vi "prosess_data.vi"(0 "Q_MotorCmd_IN":refnum<queue>, 1 "Q_MotorCmd_Err_IN":errorcluster, 2 "Q_Process_Data_IN":refnum<queue>, 3 "Q_Process_Data_Err_IN":errorcluster caption="Q_Process_DATA_Err_IN", 4 "Notifier_IN":refnum<notifier>, 5 "Error_IN":errorcluster caption="Notifier Error IN", 6 "Q_DATA_IN":refnum<queue>, 8 "Q_DATA_Err_IN":errorcluster) -> (14 "Q_Process_Data_OUT":refnum<queue>, 15 "Q_Process_Data_Err_OUT":errorcluster caption="Q_Process_DATA_Err_OUT", 16 "Q_MotorCmd_OUT":refnum<queue>, 17 "Q_MotorCmd_Err_OUT":errorcluster)   [LabVIEW 2019]
uses:
  <vilib>/Platform/TimedLoop/XDataNode/timing_clust.ctl
  <vilib>/Platform/TimedLoop/XDataNode/nitl_modes.ctl
  <vilib>/Platform/TimedLoop/XDataNode/wakeup.ctl
  RT_GLOBAL.vi
  <vilib>/Platform/TimedLoop/XDataNode/XDataNode.xnode
  <vilib>/Platform/TimedLoop/XDataNode/XDNodeRunTimeDep.lvlib
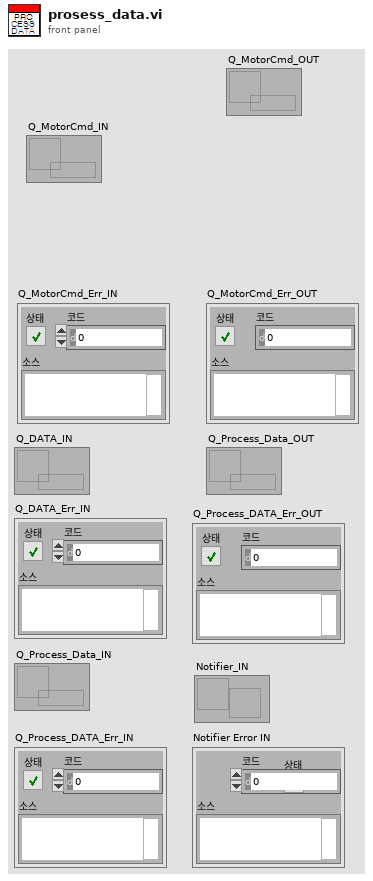
[diagram p1: front panel]
types:
  T1 = cluster{"MinPos":i32, "MaxPos":i32, "Init_Vel_UP":i32, "Init_Accel":u32, "Test_Vel":i32, "Test_Acc":u32, "Init_Onset_Load":sgl, "Init_L":bool, "Init_R":bool, "Param":cluster{"Clt_Param_L":cluster{"기준값":sgl, "검출값":sgl, "Onset_Min":sgl, "Onset_Max":sgl, "Peak_Min":sgl, "Peak_Max":sgl, "Base":i32, "Onset":i32, "Peak":i32, "Pos":i32, "Offset":sgl}, "Clt_Param_R":cluster{"기준값":sgl, "검출값":sgl, "Onset_Min":sgl, "Onset_Max":sgl, "Peak_Min":sgl, "Peak_Max":sgl, "Base":i32, "Onset":i32, "Peak":i32, "Pos":i32, "Offset":sgl}}, "Onset_Load_L":sgl, "Max_Load_L":sgl, "Onset_Load_R":sgl, "Max_Load_R":sgl, "Init_Vel_DWON":i32, "Load_Warn":sgl, "Load_Alarm":sgl}
  T2 = typedef "XDNodeRunTimeDep.lvlib/timing_clust.ctl" = cluster{"Expected End [f-1]":u64, "Actual End [f-1]":u64, "Finished Late? [f-1]":bool, "Expected End [i-1]":u64, "Actual End [i-1]":u64, "Finished Late? [i-1]":bool, "Expected Start [i]":u64, "Actual Start [i]":u64, "Expected Start [f]":u64, "Actual Start [f]":u64, "Source Name":string, "Structure Name":string, "Period":i64, "Deadline":i64, "Offset":i64, "Start":i64, "Priority":i32, "Timeout":i32, "Mode":T3, "Wakeup Reason":T4, "Error":errorcluster, "Source Type":string, "Secondary Source Type":string, "Global End Time":u64, "Global Start Time":u64, "Frame Duration":u64, "Iteration Duration":u64, "Assigned CPU":i32, "I/O Scan Engine Mode":u32}
  T3 = typedef "XDNodeRunTimeDep.lvlib/nitl_modes.ctl" = enum32{"No Change", "Process missed periods, maintain original phase", "Discard missed periods, maintain original phase", "Process missed periods, ignore original phase", "Discard missed periods, ignore original phase"}
  T4 = typedef "XDNodeRunTimeDep.lvlib/wakeup.ctl" = enum32{"Normal", "Aborted", "Asynchronous wakeup", "Timing source error", "Timed loop error", "Timeout"}
  T5 = cluster{"Num_L":u32, "Period_L":u32, "GCP_L":sgl, "Num_R":u32, "Period_R":u32, "GCP_R":sgl, "FPGA_Data":sgl[], "Status_L":cluster{"Ready to switch on":bool, "Switched on":bool, "Operation enable":bool, "Fault":bool, "Voltage enable":bool, "Quick stop":bool, "Switch on disable":bool, "not used (warning)":bool, "Offset current measured":bool, "Remote":bool, "Operation mode specific":bool, "Internal limit active":bool, "Operation mode specific":bool, "Operation mode specific":bool, "Refresh cycle of power stage":bool, "Position referenced to home position":bool}, "Status_R":cluster{"Ready to switch on":bool, "Switched on":bool, "Operation enable":bool, "Fault":bool, "Voltage enable":bool, "Quick stop":bool, "Switch on disable":bool, "not used (warning)":bool, "Offset current measured":bool, "Remote":bool, "Operation mode specific":bool, "Internal limit active":bool, "Operation mode specific":bool, "Operation mode specific":bool, "Refresh cycle of power stage":bool, "Position referenced to home position":bool}, "Pos_L":i32, "Pos_R":i32, "TargetPos_L":i32, "TargetPos_R":i32, "Flag_L":enum16{"Release_Start", "Onset_Start", "Peak_Start", "Calculate"}, "Flag_R":enum16{"Release_Start", "Onset_Start", "Peak_Start", "Calculate"}, "LOAD_CELL_PEAK_L":sgl[], "LOAD_CELL_PEAK_R":sgl[], "D_Pos_L":i32, "D_Pos_R":i32, "A_Velocity_L":i32, "A_Velocity_R":i32, "A_Current_L":i16, "A_Current_R":i16}
  T6 = cluster{"Cmd":string, "Data1":variant, "Data2":variant}
  T7 = cluster{"FPGA_Data":sgl[], "Tick":u32, "Cmd":string, "Param":variant}
  T8 = cluster{"Ready to switch on":bool, "Switched on":bool, "Operation enable":bool, "Fault":bool, "Voltage enable":bool, "Quick stop":bool, "Switch on disable":bool, "not used (warning)":bool, "Offset current measured":bool, "Remote":bool, "Operation mode specific":bool, "Internal limit active":bool, "Operation mode specific":bool, "Operation mode specific":bool, "Refresh cycle of power stage":bool, "Position referenced to home position":bool}
  T9 = enum16{"Release_Start", "Onset_Start", "Peak_Start", "Calculate"}
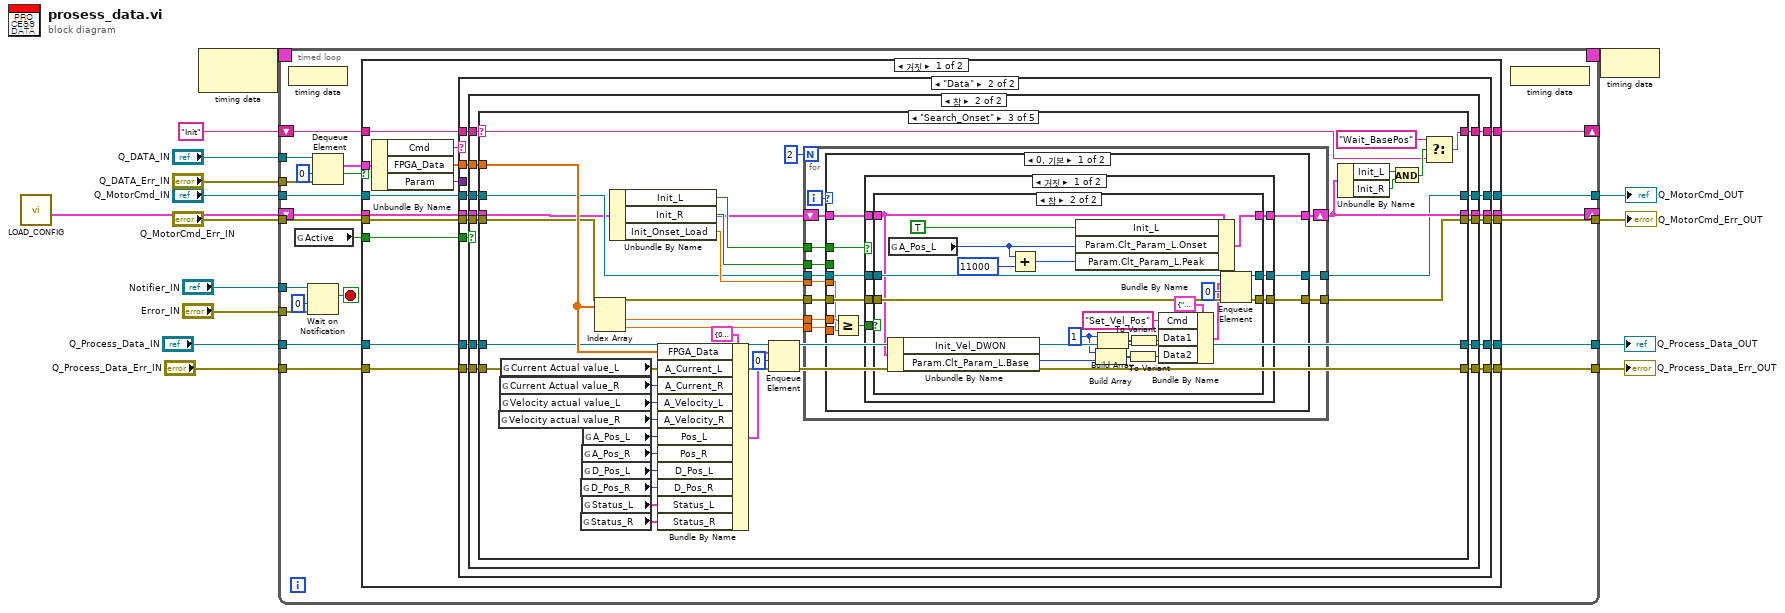
[diagram p0: block diagram]
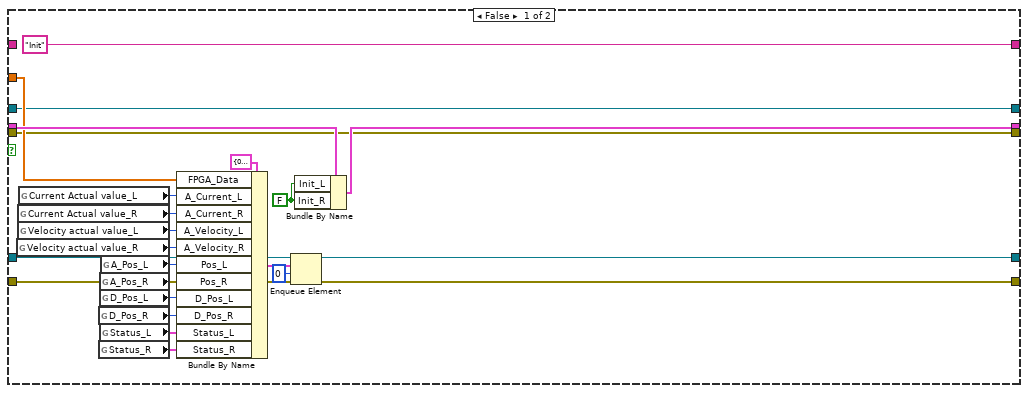
[diagram p3: hidden frame]
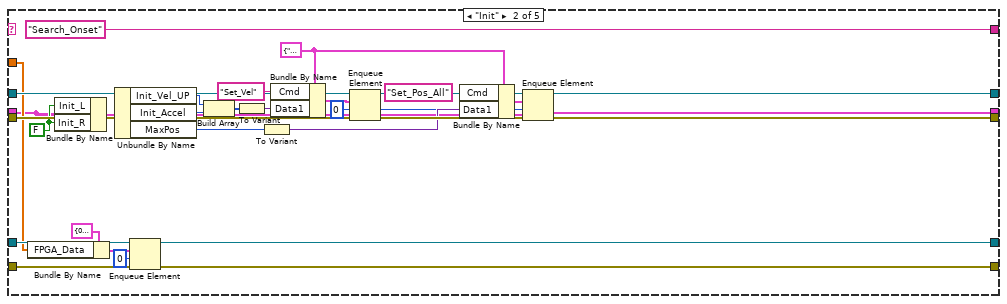
[diagram p5: hidden frame]
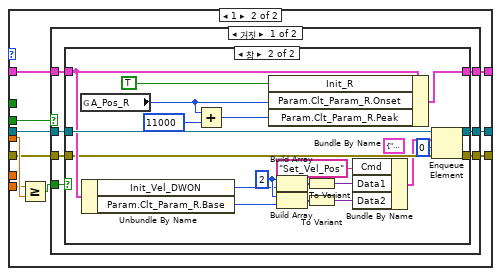
[diagram p8: hidden frame]
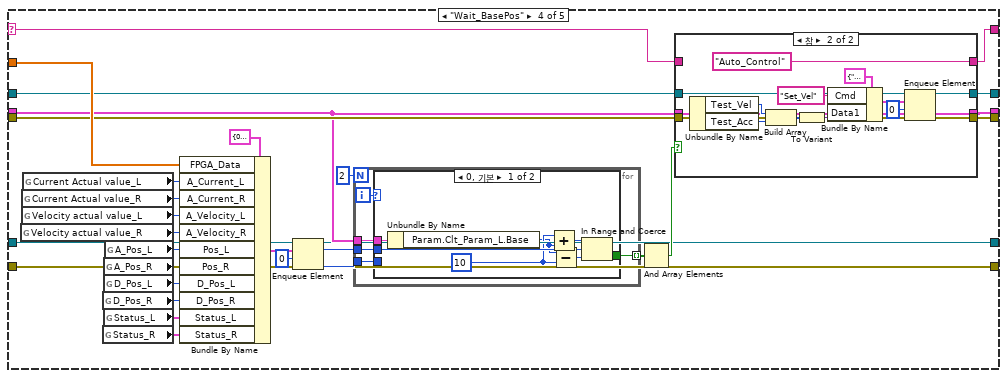
[diagram p11: hidden frame]
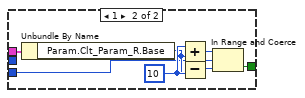
[diagram p13: hidden frame]
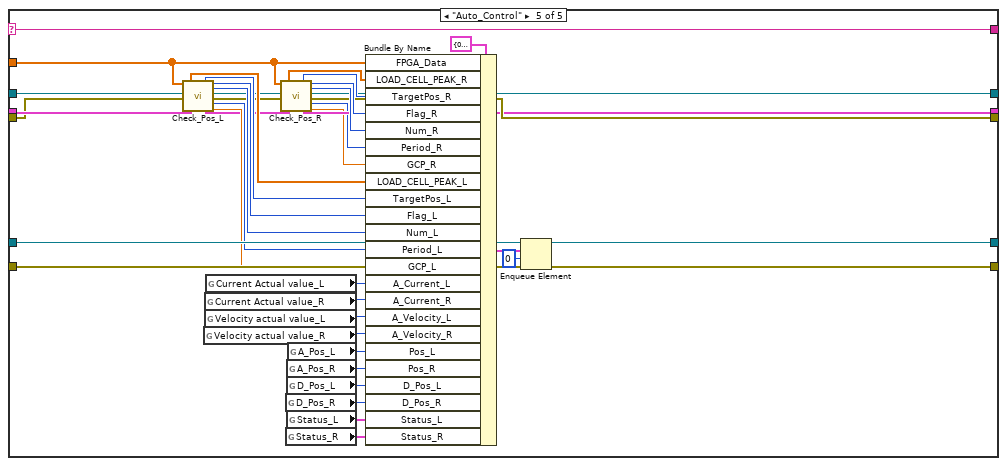
[diagram p14: hidden frame]
diagram:
  n1 = call "LOAD_CONFIG.vi"() -> ("Param_Out"=w7:T1)  [unwired: 10 in, 1 out]
  n2 = node-c288() -> (w9:T2)  [unwired: 1 in]
  n3 = timed-loop {
    shift-right: [w37] -> _
    shift-left: "Init" -> [w38]
    tunnel: "Q_DATA_IN" -> [w35]
    tunnel: "Q_DATA_Err_IN" -> [w34]
    tunnel: "Q_MotorCmd_IN" -> [w30]
    tunnel: "Q_MotorCmd_Err_IN" -> [w29]
    tunnel: "Q_Process_Data_IN" -> [w28]
    tunnel: "Q_Process_Data_Err_IN" -> [w27]
    timing: w9 -> [_]
    timing-out: [_] -> w8
    shift-right: [w25] -> _
    shift-left: w7 -> [w26]
    tunnel: "Notifier_IN" -> [w22]
    tunnel: "Error_IN" -> [w21]
    tunnel: [w20] -> w4
    tunnel: [w19] -> w3
    tunnel: [w18] -> w2
    tunnel: [w17] -> w1
    stop <- w24 stop-if-true
    n4 = node-c288() -> ()  [unwired: 1 in]
    n5 = global read "RT_GLOBAL.vi" "Active"() -> (w31:bool)
    n6 = Wait on Notification(notifier=w22, timeout in ms (-1)=0 ("타임아웃(ms) (-1)"), error in (no error)=w21) -> (notification=w24:bool)  [unwired: 1 in, 3 out]
    n7 = Dequeue Element(queue=w35, timeout in ms (-1)=0 ("타임아웃(ms) (-1)"), error in (no error)=w34) -> (element=w32:T7, timed out?=w33:bool)  [unwired: 2 out]
    n8 = case shown="거짓" w33 {
      tunnel: [w47 w398] -> w25
      tunnel: w26 -> [w54 w398]
      tunnel: w38 -> [w57 w397]
      tunnel: [w50 w397] -> w37
      tunnel: w32 -> [w56 _]
      tunnel: w31 -> [w51 _]
      tunnel: w30 -> [w49 w396]
      tunnel: w29 -> [w48 w395]
      tunnel: w28 -> [w46 w394]
      tunnel: w27 -> [w45 w393]
      tunnel: [w44 w396] -> w20
      tunnel: [w43 w395] -> w19
      tunnel: [w42 w394] -> w18
      tunnel: [w41 w393] -> w17
      frame False {
        n9 = Unbundle By Name(w56) -> ("Cmd"=w55:string, "FPGA_Data"=w52:sgl[], "Param"=w53:variant)
        n10 = case shown="\"Data\"" w55 {
          tunnel: w57 -> [w63 w77]
          tunnel: w54 -> [w62 w75]
          tunnel: w53 -> [_ _]
          tunnel: w52 -> [_ w76]
          tunnel: w51 -> [_ w74]
          tunnel: [w63 w73] -> w50
          tunnel: w49 -> [w61 w72]
          tunnel: w48 -> [w60 w71]
          tunnel: [w62 w70] -> w47
          tunnel: w46 -> [w59 w69]
          tunnel: w45 -> [w58 w68]
          tunnel: [w61 w67] -> w44
          tunnel: [w60 w66] -> w43
          tunnel: [w59 w65] -> w42
          tunnel: [w58 w64] -> w41
          frame "거짓", Default {
          }
          frame "Data" {
            n11 = case shown="참" w74 {
              tunnel: w77 -> [_ w107]
              tunnel: w76 -> [w93 w110]
              tunnel: w75 -> [w99 w113]
              tunnel: ["Init" w114] -> w73
              tunnel: w72 -> [w81 w112]
              tunnel: w71 -> [w80 w111]
              tunnel: [w98 w109] -> w70
              tunnel: w69 -> [w95 w108]
              tunnel: w68 -> [w94 w106]
              tunnel: [w81 w105] -> w67
              tunnel: [w80 w104] -> w66
              tunnel: [w79 w103] -> w65
              tunnel: [w78 w102] -> w64
              frame False {
                w100 = FALSE ("Init_L")
                n12 = global read "RT_GLOBAL.vi" "Velocity actual value_R"() -> (w88:i32)
                n13 = global read "RT_GLOBAL.vi" "Current Actual value_R"() -> (w90:i16)
                n14 = global read "RT_GLOBAL.vi" "Velocity actual value_L"() -> (w89:i32)
                n15 = global read "RT_GLOBAL.vi" "Current Actual value_L"() -> (w91:i16)
                n16 = global read "RT_GLOBAL.vi" "D_Pos_R"() -> (w84:i32)
                n17 = global read "RT_GLOBAL.vi" "Status_R"() -> (w82:T8)
                n18 = global read "RT_GLOBAL.vi" "A_Pos_R"() -> (w86:i32)
                n19 = global read "RT_GLOBAL.vi" "D_Pos_L"() -> (w85:i32)
                n20 = global read "RT_GLOBAL.vi" "Status_L"() -> (w83:T8)
                n21 = global read "RT_GLOBAL.vi" "A_Pos_L"() -> (w87:i32)
                n22 = Bundle By Name(cluster=T5 {"Num_L"=0, "Period_L"=0, "GCP_L"=0.0, "Num_R"=0, "Period_R"=0, "GCP_R"=0.0, "FPGA_Data"=[], "Status_L"={"Ready to switch on"=TRUE, "Switched on"=TRUE, "Operation enable"=TRUE, "Fault"=FALSE, "Voltage enable"=TRUE, "Quick stop"=TRUE, "Switch on disable"=FALSE, "not used (warning)"=FALSE, "Offset current measured"=FALSE, "Remote"=TRUE, "Operation mode specific"=TRUE, "Internal limit active"=FALSE, "Operation mode specific"=FALSE, "Operation mode specific"=FALSE, "Refresh cycle of power stage"=FALSE, "Position referenced to home position"=FALSE}, "Status_R"={"Ready to switch on"=TRUE, "Switched on"=TRUE, "Operation enable"=TRUE, "Fault"=FALSE, "Voltage enable"=TRUE, "Quick stop"=TRUE, "Switch on disable"=FALSE, "not used (warning)"=FALSE, "Offset current measured"=FALSE, "Remote"=TRUE, "Operation mode specific"=TRUE, "Internal limit active"=FALSE, "Operation mode specific"=FALSE, "Operation mode specific"=FALSE, "Refresh cycle of power stage"=FALSE, "Position referenced to home position"=FALSE}, "Pos_L"=0, "Pos_R"=0, "TargetPos_L"=0, "TargetPos_R"=0, "Flag_L"=enum."Release_Start", "Flag_R"=enum."Release_Start", "LOAD_CELL_PEAK_L"=[12.0, 8.0], "LOAD_CELL_PEAK_R"=[], "D_Pos_L"=0, "D_Pos_R"=0, "A_Velocity_L"=0, "A_Velocity_R"=0, "A_Current_L"=0, "A_Current_R"=0}, "FPGA_Data"=w93, "A_Current_L"=w91, "A_Current_R"=w90, "A_Velocity_L"=w89, "A_Velocity_R"=w88, "Pos_L"=w87, "Pos_R"=w86, "D_Pos_L"=w85, "D_Pos_R"=w84, "Status_L"=w83, "Status_R"=w82) -> (w97:T5)
                n23 = Enqueue Element(queue=w95, element=w97, timeout in ms (-1)=0 ("타임아웃(ms) (-1)"), error in (no error)=w94) -> (queue out=w79:refnum<queue>, error out=w78:errorcluster)  [unwired: 1 out]
                n24 = Bundle By Name(cluster=w99, "Init_L"=w100, "Init_R"=w100) -> (w98:T1)
              }
              frame True {
                n25 = case shown="\"Search_Onset\"" w107 {
                  selector: w107 -> [w120 _ w172 w297 w389]
                  tunnel: [w120 "Search_Onset" w173 w292 w389] -> w114
                  tunnel: w113 -> [w119 w128 w155 w293 w373]
                  tunnel: w112 -> [w118 w149 w170 w294 w368]
                  tunnel: w111 -> [w117 w148 w169 w295 w369]
                  tunnel: w110 -> [_ w143 w182 w314 w365]
                  tunnel: [w119 w129 w171 w287 w357] -> w109
                  tunnel: w108 -> [w116 w145 w180 w311 w391]
                  tunnel: w106 -> [w115 w144 w179 w310 w388]
                  tunnel: [w118 w124 w154 w291 w360] -> w105
                  tunnel: [w117 w123 w153 w290 w359] -> w104
                  tunnel: [w116 w122 w152 w289 w354] -> w103
                  tunnel: [w115 w121 w151 w288 w353] -> w102
                  frame "거짓", Default {
                  }
                  frame "Init" {
                    w133 = T6 {"Cmd"="", "Data1"=variant, "Data2"=variant}
                    w134 = FALSE ("Init_L")
                    w130 = 0 ("타임아웃(ms) (-1)")
                    n26 = Bundle By Name(cluster=T5 {"Num_L"=0, "Period_L"=0, "GCP_L"=0.0, "Num_R"=0, "Period_R"=0, "GCP_R"=0.0, "FPGA_Data"=[], "Status_L"={"Ready to switch on"=TRUE, "Switched on"=TRUE, "Operation enable"=TRUE, "Fault"=FALSE, "Voltage enable"=TRUE, "Quick stop"=TRUE, "Switch on disable"=FALSE, "not used (warning)"=FALSE, "Offset current measured"=FALSE, "Remote"=TRUE, "Operation mode specific"=TRUE, "Internal limit active"=FALSE, "Operation mode specific"=FALSE, "Operation mode specific"=FALSE, "Refresh cycle of power stage"=FALSE, "Position referenced to home position"=FALSE}, "Status_R"={"Ready to switch on"=TRUE, "Switched on"=TRUE, "Operation enable"=TRUE, "Fault"=FALSE, "Voltage enable"=TRUE, "Quick stop"=TRUE, "Switch on disable"=FALSE, "not used (warning)"=FALSE, "Offset current measured"=FALSE, "Remote"=TRUE, "Operation mode specific"=TRUE, "Internal limit active"=FALSE, "Operation mode specific"=FALSE, "Operation mode specific"=FALSE, "Refresh cycle of power stage"=FALSE, "Position referenced to home position"=FALSE}, "Pos_L"=0, "Pos_R"=0, "TargetPos_L"=0, "TargetPos_R"=0, "Flag_L"=enum."Release_Start", "Flag_R"=enum."Release_Start", "LOAD_CELL_PEAK_L"=[12.0, 8.0], "LOAD_CELL_PEAK_R"=[], "D_Pos_L"=0, "D_Pos_R"=0, "A_Velocity_L"=0, "A_Velocity_R"=0, "A_Current_L"=0, "A_Current_R"=0}, "FPGA_Data"=w143) -> (w147:T5)
                    n27 = Bundle By Name(cluster=w128, "Init_L"=w134, "Init_R"=w134) -> (w129:T1)
                    n28 = Unbundle By Name(w128) -> ("Init_Vel_UP"=w127:i32, "Init_Accel"=w126:u32, "MaxPos"=w125:i32)
                    n29 = Enqueue Element(queue=w145, element=w147, timeout in ms (-1)=0 ("타임아웃(ms) (-1)"), error in (no error)=w144) -> (queue out=w122:refnum<queue>, error out=w121:errorcluster)  [unwired: 1 out]
                    n30 = Build Array(w127, w126) -> (w139:u32[])
                    n31 = To Variant(anything=w139) -> (Variant=w140:variant)
                    n32 = To Variant(anything=w125) -> (Variant=w135:variant)
                    n33 = Bundle By Name(cluster=w133, "Cmd"="Set_Vel", "Data1"=w140) -> (w132:T6)
                    n34 = Enqueue Element(queue=w149, element=w132, timeout in ms (-1)=w130, error in (no error)=w148) -> (queue out=w138:refnum<queue>, error out=w137:errorcluster)  [unwired: 1 out]
                    n35 = Bundle By Name(cluster=w133, "Cmd"="Set_Pos_All", "Data1"=w135) -> (w131:T6)
                    n36 = Enqueue Element(queue=w138, element=w131, timeout in ms (-1)=w130, error in (no error)=w137) -> (queue out=w124:refnum<queue>, error out=w123:errorcluster)  [unwired: 1 out]
                  }
                  frame "Search_Onset" {
                    n37 = global read "RT_GLOBAL.vi" "Velocity actual value_R"() -> (w164:i32)
                    n38 = global read "RT_GLOBAL.vi" "Current Actual value_R"() -> (w166:i16)
                    n39 = global read "RT_GLOBAL.vi" "Velocity actual value_L"() -> (w165:i32)
                    n40 = global read "RT_GLOBAL.vi" "Current Actual value_L"() -> (w167:i16)
                    n41 = global read "RT_GLOBAL.vi" "D_Pos_R"() -> (w160:i32)
                    n42 = global read "RT_GLOBAL.vi" "Status_R"() -> (w158:T8)
                    n43 = global read "RT_GLOBAL.vi" "A_Pos_R"() -> (w162:i32)
                    n44 = global read "RT_GLOBAL.vi" "D_Pos_L"() -> (w161:i32)
                    n45 = global read "RT_GLOBAL.vi" "Status_L"() -> (w159:T8)
                    n46 = global read "RT_GLOBAL.vi" "A_Pos_L"() -> (w163:i32)
                    n47 = Index Array(array=w182) -> (element #1=w157:sgl, element #2=w156:sgl)  [unwired: 2 in]
                    n48 = Unbundle By Name(w155) -> ("Init_L"=w185:bool, "Init_R"=w184:bool, "Init_Onset_Load"=w183:sgl)
                    n49 = Bundle By Name(cluster=T5 {"Num_L"=0, "Period_L"=0, "GCP_L"=0.0, "Num_R"=0, "Period_R"=0, "GCP_R"=0.0, "FPGA_Data"=[], "Status_L"={"Ready to switch on"=TRUE, "Switched on"=TRUE, "Operation enable"=TRUE, "Fault"=FALSE, "Voltage enable"=TRUE, "Quick stop"=TRUE, "Switch on disable"=FALSE, "not used (warning)"=FALSE, "Offset current measured"=FALSE, "Remote"=TRUE, "Operation mode specific"=TRUE, "Internal limit active"=FALSE, "Operation mode specific"=FALSE, "Operation mode specific"=FALSE, "Refresh cycle of power stage"=FALSE, "Position referenced to home position"=FALSE}, "Status_R"={"Ready to switch on"=TRUE, "Switched on"=TRUE, "Operation enable"=TRUE, "Fault"=FALSE, "Voltage enable"=TRUE, "Quick stop"=TRUE, "Switch on disable"=FALSE, "not used (warning)"=FALSE, "Offset current measured"=FALSE, "Remote"=TRUE, "Operation mode specific"=TRUE, "Internal limit active"=FALSE, "Operation mode specific"=FALSE, "Operation mode specific"=FALSE, "Refresh cycle of power stage"=FALSE, "Position referenced to home position"=FALSE}, "Pos_L"=0, "Pos_R"=0, "TargetPos_L"=0, "TargetPos_R"=0, "Flag_L"=enum."Release_Start", "Flag_R"=enum."Release_Start", "LOAD_CELL_PEAK_L"=[12.0, 8.0], "LOAD_CELL_PEAK_R"=[], "D_Pos_L"=0, "D_Pos_R"=0, "A_Velocity_L"=0, "A_Velocity_R"=0, "A_Current_L"=0, "A_Current_R"=0}, "FPGA_Data"=w182, "A_Current_L"=w167, "A_Current_R"=w166, "A_Velocity_L"=w165, "A_Velocity_R"=w164, "Pos_L"=w163, "Pos_R"=w162, "D_Pos_L"=w161, "D_Pos_R"=w160, "Status_L"=w159, "Status_R"=w158) -> (w178:T5)
                    n50 = Enqueue Element(queue=w180, element=w178, timeout in ms (-1)=0 ("타임아웃(ms) (-1)"), error in (no error)=w179) -> (queue out=w152:refnum<queue>, error out=w151:errorcluster)  [unwired: 1 out]
                    n51 = for {
                      N: 2 -> [_]
                      shift-right: [w191] -> w171
                      shift-left: w155 -> [w197]
                      tunnel: w185 -> [w196]
                      tunnel: w184 -> [w195]
                      tunnel: w183 -> [w194]
                      tunnel: w170 -> [w193]
                      tunnel: w169 -> [w192]
                      tunnel: w157 -> [w190]
                      tunnel: w156 -> [w189]
                      tunnel: [w188] -> w154
                      tunnel: [w187] -> w153
                      i -> [w198]
                      n52 = case shown="0, 기본" w198 {
                        tunnel: w197 -> [w207 w251]
                        tunnel: w196 -> [w204 _]
                        tunnel: w195 -> [_ w248]
                        tunnel: w194 -> [w201 w252]
                        tunnel: w193 -> [w206 w249]
                        tunnel: w192 -> [w205 w246]
                        tunnel: w190 -> [w202 _]
                        tunnel: [w208 w250] -> w191
                        tunnel: w189 -> [_ w245]
                        tunnel: [w200 w244] -> w188
                        tunnel: [w199 w243] -> w187
                        frame 0, Default {
                          n53 = Greater Or Equal?(x=w202, y=w201) -> (x >= y?=w203:bool)
                          n54 = case shown="거짓" w204 {
                            tunnel: [w215 w242] -> w208
                            tunnel: w207 -> [w214 w242]
                            tunnel: w206 -> [w213 w241]
                            tunnel: w205 -> [w212 w240]
                            tunnel: w203 -> [w211 _]
                            tunnel: [w210 w241] -> w200
                            tunnel: [w209 w240] -> w199
                            frame False {
                              n55 = case shown="참" w211 {
                                tunnel: [w218 w234] -> w215
                                tunnel: w214 -> [w218 w230]
                                tunnel: w213 -> [w217 w233]
                                tunnel: w212 -> [w216 w232]
                                tunnel: [w217 w220] -> w210
                                tunnel: [w216 w219] -> w209
                                frame False {
                                }
                                frame True {
                                w222 = 1 ("원소")
                                n56 = Unbundle By Name(w230) -> ("Init_Vel_DWON"=w224:i32, "Param.Clt_Param_L.Base"=w221:i32)
                                n57 = global read "RT_GLOBAL.vi" "A_Pos_L"() -> (w226:i32)
                                n58 = Add(x=w226, y=11000) -> (x+y=w227:i32)
                                n59 = Bundle By Name(cluster=w230, "Init_L"=TRUE, "Param.Clt_Param_L.Onset"=w226, "Param.Clt_Param_L.Peak"=w227) -> (w234:T1)
                                n60 = Build Array(w222, w221) -> (w235:i32[])
                                n61 = Build Array(w222, w224) -> (w237:i32[])
                                n62 = To Variant(anything=w235) -> (Variant=w223:variant)
                                n63 = To Variant(anything=w237) -> (Variant=w239:variant)
                                n64 = Bundle By Name(cluster=T6 {"Cmd"="", "Data1"=variant, "Data2"=variant}, "Cmd"="Set_Vel_Pos", "Data1"=w239, "Data2"=w223) -> (w228:T6)
                                n65 = Enqueue Element(queue=w233, element=w228, timeout in ms (-1)=0 ("타임아웃(ms) (-1)"), error in (no error)=w232) -> (queue out=w220:refnum<queue>, error out=w219:errorcluster)  [unwired: 1 out]
                                }
                              }
                            }
                            frame True {
                            }
                          }
                        }
                        frame 1 {
                          n66 = Greater Or Equal?(x=w245, y=w252) -> (x >= y?=w247:bool)
                          n67 = case shown="거짓" w248 {
                            tunnel: w251 -> [w257 w286]
                            tunnel: [w259 w286] -> w250
                            tunnel: w249 -> [w258 w285]
                            tunnel: w247 -> [w256 _]
                            tunnel: w246 -> [w255 w284]
                            tunnel: [w254 w285] -> w244
                            tunnel: [w253 w284] -> w243
                            frame False {
                              n68 = case shown="참" w256 {
                                tunnel: [w262 w282] -> w259
                                tunnel: w258 -> [w261 w280]
                                tunnel: w257 -> [w262 w279]
                                tunnel: w255 -> [w260 w274]
                                tunnel: [w261 w264] -> w254
                                tunnel: [w260 w263] -> w253
                                frame False {
                                }
                                frame True {
                                w270 = 2 ("원소")
                                n69 = global read "RT_GLOBAL.vi" "A_Pos_R"() -> (w268:i32)
                                n70 = Unbundle By Name(w279) -> ("Init_Vel_DWON"=w266:i32, "Param.Clt_Param_R.Base"=w265:i32)
                                n71 = Add(x=w268, y=11000) -> (x+y=w269:i32)
                                n72 = Bundle By Name(cluster=w279, "Init_R"=TRUE ("Init_L"), "Param.Clt_Param_R.Onset"=w268, "Param.Clt_Param_R.Peak"=w269) -> (w282:T1)
                                n73 = Build Array(w270, w266) -> (w276:i32[])
                                n74 = Build Array(w270, w265) -> (w275:i32[])
                                n75 = To Variant(anything=w276) -> (Variant=w278:variant)
                                n76 = To Variant(anything=w275) -> (Variant=w271:variant)
                                n77 = Bundle By Name(cluster=T6 {"Cmd"="", "Data1"=variant, "Data2"=variant}, "Cmd"="Set_Vel_Pos", "Data1"=w278, "Data2"=w271) -> (w272:T6)
                                n78 = Enqueue Element(queue=w280, element=w272, timeout in ms (-1)=0 ("타임아웃(ms) (-1)"), error in (no error)=w274) -> (queue out=w264:refnum<queue>, error out=w263:errorcluster)  [unwired: 1 out]
                                }
                              }
                            }
                            frame True {
                            }
                          }
                        }
                      }
                    }
                    n79 = Unbundle By Name(w171) -> ("Init_L"=w177:bool, "Init_R"=w176:bool)
                    n80 = And(x=w177, y=w176) -> (x .and. y?=w175:bool)
                    n81 = Select(t="Wait_BasePos", s=w175, f=w172) -> (s? t:f=w173:string)
                  }
                  frame "Wait_BasePos" {
                    n82 = global read "RT_GLOBAL.vi" "Velocity actual value_R"() -> (w305:i32)
                    n83 = global read "RT_GLOBAL.vi" "Current Actual value_R"() -> (w307:i16)
                    n84 = global read "RT_GLOBAL.vi" "Velocity actual value_L"() -> (w306:i32)
                    n85 = global read "RT_GLOBAL.vi" "Current Actual value_L"() -> (w308:i16)
                    n86 = global read "RT_GLOBAL.vi" "D_Pos_R"() -> (w303:i32)
                    n87 = global read "RT_GLOBAL.vi" "Status_R"() -> (w301:T8)
                    n88 = global read "RT_GLOBAL.vi" "A_Pos_R"() -> (w299:i32)
                    n89 = global read "RT_GLOBAL.vi" "D_Pos_L"() -> (w304:i32)
                    n90 = global read "RT_GLOBAL.vi" "Status_L"() -> (w302:T8)
                    n91 = global read "RT_GLOBAL.vi" "A_Pos_L"() -> (w300:i32)
                    n92 = Bundle By Name(cluster=T5 {"Num_L"=0, "Period_L"=0, "GCP_L"=0.0, "Num_R"=0, "Period_R"=0, "GCP_R"=0.0, "FPGA_Data"=[], "Status_L"={"Ready to switch on"=TRUE, "Switched on"=TRUE, "Operation enable"=TRUE, "Fault"=FALSE, "Voltage enable"=TRUE, "Quick stop"=TRUE, "Switch on disable"=FALSE, "not used (warning)"=FALSE, "Offset current measured"=FALSE, "Remote"=TRUE, "Operation mode specific"=TRUE, "Internal limit active"=FALSE, "Operation mode specific"=FALSE, "Operation mode specific"=FALSE, "Refresh cycle of power stage"=FALSE, "Position referenced to home position"=FALSE}, "Status_R"={"Ready to switch on"=TRUE, "Switched on"=TRUE, "Operation enable"=TRUE, "Fault"=FALSE, "Voltage enable"=TRUE, "Quick stop"=TRUE, "Switch on disable"=FALSE, "not used (warning)"=FALSE, "Offset current measured"=FALSE, "Remote"=TRUE, "Operation mode specific"=TRUE, "Internal limit active"=FALSE, "Operation mode specific"=FALSE, "Operation mode specific"=FALSE, "Refresh cycle of power stage"=FALSE, "Position referenced to home position"=FALSE}, "Pos_L"=0, "Pos_R"=0, "TargetPos_L"=0, "TargetPos_R"=0, "Flag_L"=enum."Release_Start", "Flag_R"=enum."Release_Start", "LOAD_CELL_PEAK_L"=[12.0, 8.0], "LOAD_CELL_PEAK_R"=[], "D_Pos_L"=0, "D_Pos_R"=0, "A_Velocity_L"=0, "A_Velocity_R"=0, "A_Current_L"=0, "A_Current_R"=0}, "FPGA_Data"=w314, "A_Current_L"=w308, "A_Current_R"=w307, "A_Velocity_L"=w306, "A_Velocity_R"=w305, "Pos_L"=w300, "Pos_R"=w299, "D_Pos_L"=w304, "D_Pos_R"=w303, "Status_L"=w302, "Status_R"=w301) -> (w315:T5)
                    n93 = Enqueue Element(queue=w311, element=w315, timeout in ms (-1)=0 ("타임아웃(ms) (-1)"), error in (no error)=w310) -> (queue out=w289:refnum<queue>, error out=w288:errorcluster)  [unwired: 1 out]
                    n94 = for {
                      N: 2 -> [_]
                      tunnel: w293 -> [w337]
                      tunnel: [w336] -> w312 mode=indexing
                      tunnel: w300 -> [w335]
                      tunnel: w299 -> [w334]
                      i -> [w338]
                      n95 = case shown="0, 기본" w338 {
                        tunnel: w335 -> [w345 _]
                        tunnel: w337 -> [w340 w348]
                        tunnel: [w339 w347] -> w336
                        tunnel: w334 -> [_ w346]
                        frame 0, Default {
                          w344 = 10 ("x")
                          n96 = Unbundle By Name(w340) -> ("Param.Clt_Param_L.Base"=w343:i32)
                          n97 = Add(x=w344, y=w343) -> (x+y=w341:i32)
                          n98 = Subtract(x=w343, y=w344) -> (x-y=w342:i32)
                          n99 = In Range and Coerce(upper limit=w341, x=w345, lower limit=w342) -> (In Range?=w339:bool)  [unwired: 1 out]
                        }
                        frame 1 {
                          w352 = 10 ("x")
                          n100 = Unbundle By Name(w348) -> ("Param.Clt_Param_R.Base"=w351:i32)
                          n101 = Add(x=w352, y=w351) -> (x+y=w349:i32)
                          n102 = Subtract(x=w351, y=w352) -> (x-y=w350:i32)
                          n103 = In Range and Coerce(upper limit=w349, x=w346, lower limit=w350) -> (In Range?=w347:bool)  [unwired: 1 out]
                        }
                      }
                    }
                    n104 = And Array Elements(Boolean array=w312) -> (logical AND=w296:bool)
                    n105 = case shown="참" w296 {
                      tunnel: w293 -> [w319 w324]
                      tunnel: [w319 w324] -> w287
                      tunnel: [w318 "Auto_Control"] -> w292
                      tunnel: w297 -> [w318 _]
                      tunnel: w294 -> [w317 w326]
                      tunnel: w295 -> [w316 w325]
                      tunnel: [w317 w321] -> w291
                      tunnel: [w316 w320] -> w290
                      frame False {
                      }
                      frame True {
                        n106 = Unbundle By Name(w324) -> ("Test_Vel"=w331:i32, "Test_Acc"=w332:u32)
                        n107 = Build Array(w331, w332) -> (w330:u32[])
                        n108 = To Variant(anything=w330) -> (Variant=w329:variant)
                        n109 = Bundle By Name(cluster=T6 {"Cmd"="", "Data1"=variant, "Data2"=variant}, "Cmd"="Set_Vel", "Data1"=w329) -> (w322:T6)
                        n110 = Enqueue Element(queue=w326, element=w322, timeout in ms (-1)=0 ("타임아웃(ms) (-1)"), error in (no error)=w325) -> (queue out=w321:refnum<queue>, error out=w320:errorcluster)  [unwired: 1 out]
                      }
                    }
                  }
                  frame "Auto_Control" {
                    n111 = call "Check_Pos_L.vi"("FPGA_Data"=w365, "Q_MotorCmd_IN"=w368, "Q_MotorCmd_Err_IN"=w369, "Param_In"=w373) -> ("LOAD_CELL_PEAK_L"=w376:sgl[], "Target_Pos"=w370:i32, "Param_Out"=w358:T1, "Flag"=w375:T9, "L_NUM"=w374:u32, "Q_MotorCmd_OUT"=w367:refnum<queue>, "Q_MotorCmd_Err_OUT"=w366:errorcluster, "L_Period"=w371:u32, "L_GCP"=w372:sgl)  [unwired: 7 in]
                    n112 = global read "RT_GLOBAL.vi" "Velocity actual value_R"() -> (w383:i32)
                    n113 = global read "RT_GLOBAL.vi" "Current Actual value_R"() -> (w385:i16)
                    n114 = global read "RT_GLOBAL.vi" "Velocity actual value_L"() -> (w384:i32)
                    n115 = global read "RT_GLOBAL.vi" "Current Actual value_L"() -> (w386:i16)
                    n116 = call "Check_Pos_R.vi"("FPGA_Data"=w365, "Q_MotorCmd_IN"=w367, "Q_MotorCmd_Err_IN"=w366, "Param_In"=w358) -> ("LOAD_CELL_PEAK_R"=w364:sgl[], "Target_Pos"=w363:i32, "Param_Out"=w357:T1, "Flag"=w362:T9, "R_NUM"=w361:u32, "Q_MotorCmd_OUT"=w360:refnum<queue>, "Q_MotorCmd_Err_OUT"=w359:errorcluster, "R_Period"=w356:u32, "R_GCP"=w355:sgl)  [unwired: 7 in]
                    n117 = global read "RT_GLOBAL.vi" "D_Pos_R"() -> (w379:i32)
                    n118 = global read "RT_GLOBAL.vi" "Status_R"() -> (w377:T8)
                    n119 = global read "RT_GLOBAL.vi" "A_Pos_R"() -> (w381:i32)
                    n120 = global read "RT_GLOBAL.vi" "D_Pos_L"() -> (w380:i32)
                    n121 = global read "RT_GLOBAL.vi" "Status_L"() -> (w378:T8)
                    n122 = global read "RT_GLOBAL.vi" "A_Pos_L"() -> (w382:i32)
                    n123 = Bundle By Name(cluster=T5 {"Num_L"=0, "Period_L"=0, "GCP_L"=0.0, "Num_R"=0, "Period_R"=0, "GCP_R"=0.0, "FPGA_Data"=[], "Status_L"={"Ready to switch on"=TRUE, "Switched on"=TRUE, "Operation enable"=TRUE, "Fault"=FALSE, "Voltage enable"=TRUE, "Quick stop"=TRUE, "Switch on disable"=FALSE, "not used (warning)"=FALSE, "Offset current measured"=FALSE, "Remote"=TRUE, "Operation mode specific"=TRUE, "Internal limit active"=FALSE, "Operation mode specific"=FALSE, "Operation mode specific"=FALSE, "Refresh cycle of power stage"=FALSE, "Position referenced to home position"=FALSE}, "Status_R"={"Ready to switch on"=TRUE, "Switched on"=TRUE, "Operation enable"=TRUE, "Fault"=FALSE, "Voltage enable"=TRUE, "Quick stop"=TRUE, "Switch on disable"=FALSE, "not used (warning)"=FALSE, "Offset current measured"=FALSE, "Remote"=TRUE, "Operation mode specific"=TRUE, "Internal limit active"=FALSE, "Operation mode specific"=FALSE, "Operation mode specific"=FALSE, "Refresh cycle of power stage"=FALSE, "Position referenced to home position"=FALSE}, "Pos_L"=0, "Pos_R"=0, "TargetPos_L"=0, "TargetPos_R"=0, "Flag_L"=enum."Release_Start", "Flag_R"=enum."Release_Start", "LOAD_CELL_PEAK_L"=[12.0, 8.0], "LOAD_CELL_PEAK_R"=[], "D_Pos_L"=0, "D_Pos_R"=0, "A_Velocity_L"=0, "A_Velocity_R"=0, "A_Current_L"=0, "A_Current_R"=0}, "FPGA_Data"=w365, "LOAD_CELL_PEAK_R"=w364, "TargetPos_R"=w363, "Flag_R"=w362, "Num_R"=w361, "Period_R"=w356, "GCP_R"=w355, "LOAD_CELL_PEAK_L"=w376, "TargetPos_L"=w370, "Flag_L"=w375, "Num_L"=w374, "Period_L"=w371, "GCP_L"=w372, "A_Current_L"=w386, "A_Current_R"=w385, "A_Velocity_L"=w384, "A_Velocity_R"=w383, "Pos_L"=w382, "Pos_R"=w381, "D_Pos_L"=w380, "D_Pos_R"=w379, "Status_L"=w378, "Status_R"=w377) -> (w390:T5)
                    n124 = Enqueue Element(queue=w391, element=w390, timeout in ms (-1)=0 ("타임아웃(ms) (-1)"), error in (no error)=w388) -> (queue out=w354:refnum<queue>, error out=w353:errorcluster)  [unwired: 1 out]
                  }
                }
              }
            }
          }
        }
      }
      frame True {
      }
    }
    n125 = node-c288() -> ()  [unwired: 1 out]
  }
  "Q_Process_Data_Err_OUT" <- w1
  "Q_MotorCmd_Err_OUT" <- w3
  "Q_Process_Data_OUT" <- w2
  "Q_MotorCmd_OUT" <- w4
  n126 = node-c288(w8) -> ()
